vi "pathPlanningVSS.vi"(8 "error in (no error) 2":errorcluster, 9 "Line?":bool, 11 "Game in 2":refnum<class "Game.lvclass">) -> (0 "error out 2":errorcluster, 3 "Game out 2":refnum<class "Game.lvclass">)   [LabVIEW 2023, in "Game.lvclass"]
uses:
  Game.lvclass
  Game.lvclass/Game.ctl
  Read Parameters.lvclass.vi
  Parameters_class/Parameters.lvclass
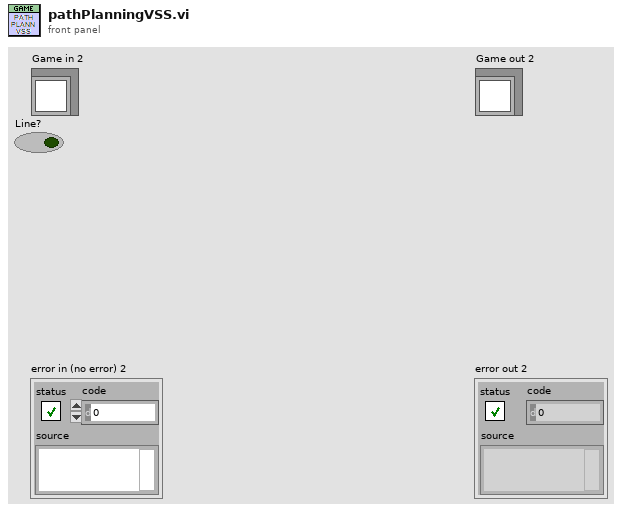
[diagram p1: front panel]
types:
  T1 = typedef "AI Input.ctl" = cluster{"our_robots":T2[], "enemy_robots":T2[], "balls":T8[], "geometry":T9, "IA Judge":T10, "Received Timestamp":timestamp, "Events":T12}
  T2 = typedef "AI Robot.ctl" = cluster{"id":u32, "function":T3, "x":dbl, "y":dbl, "orientation":dbl, "v_tangent":dbl, "v_normal":dbl, "v_ang":dbl, "kick_x":dbl, "kick_z":dbl, "dribble":bool, "Timestamp":timestamp, "estimatives":cluster{"est_v_tangent":dbl, "est_v_normal":dbl, "est_vx":dbl, "est_vy":dbl, "Pos Robot Est":dbl[]}, "dest_x_kick":dbl, "dest_y_kick":dbl, "Gap Coord":dbl[], "States":T4, "Path ":dbl[][], "Path  Smooth":dbl[][], "Dest":T5, "vx_desired":dbl, "vy_desired":dbl, "slowBehavior":bool, "VSSStates":T7}
  T3 = typedef "Functions Enum.ctl" = enum16{"2nd Striker", "Attacker", "Goalie", "Defender", "Striker", "Goto 0", "Dummy", "Kicker", "ZigZag 0", "ZigZag 1", "ZigZag 2", "ZigZag 3", "ZigZag 4", "ZigZag 5", "ZigZag 6", "ZigZag 7", "ZigZag 8", ""}
  T4 = typedef "AttackerStates.ctl" = enum16{"Pass", "GoToTangent", "BallGetting", "GoToKick", ""}
  T5 = typedef "PathDests.ctl" = T6[]
  T6 = typedef "PathDest.ctl" = cluster{"dest_x":dbl, "dest_y":dbl, "dest_orientation":dbl, "dest_vel":dbl}
  T7 = typedef "VSSAttackerStates.ctl" = enum16{"Pass", "GoToTangent", "BallGetting", "GoToKick", "Rotate anti-clockwise", "Rotate Clockwise", ""}
  T8 = typedef "AI Ball.ctl" = cluster{"x":dbl, "y":dbl, "timestamp":timestamp, "Vel_x":dbl, "Vel_y":dbl, "Pos Bola Est":dbl[], "Valid":bool}
  T9 = typedef "Field Size.ctl" = cluster{"line_width":u32, "field_length":u32, "field_width":u32, "boundary_width":u32, "referee_width":u32, "goal_width":u32, "goal_depth":u32, "goal_wall_width":u32, "center_circle_radius":u32, "defense_radius":u32, "defense_stretch":u32, "free_kick_from_defense_dist":u32, "penalty_spot_from_field_line_dist":u32, "penalty_line_from_spot_dist":u32}
  T10 = typedef "AI Judge.ctl" = cluster{"stage":string, "command":string, "our_goalie_id":dbl, "enemy_goalie_id":dbl, "command enum":T11, "Time":enum16{"Azul", "Amarelo"}}
  T11 = typedef "Command Enum.ctl" = enum16{"Halt", "Stop", "Force Start", "PKA Normal Start", "Prepare Kickoff Ally", "PKE Normal Start", "Prepare Kickoff Enemy", "Prepare Penalty Ally", "PPA Normal Start", "Prepare Penalty Enemy", "PPE Normal Start", "Direct Free Enemy", "Direct Free Ally", "Indirect Free Enemy", "Indirect Free Ally", "Timeout Enemy", "Timeout Ally", "Goal Enemy", "Goal Ally", "Ball Placement Enemy", "Ball Placement Ally", "Normal Half Time", "Extra Time Break", "Extra Half Time", "None", "Post Game"}
  T12 = typedef "Events.ctl" = cluster{"Touch":bool, "Ball out":bool, "id touch":dbl, "Ball out of \nVision":bool, "Ball inside \nGoalie area":bool, "Robot not responding":bool, "Robots responding status":dbl[], "Enemy Ball \nPossession":bool, "Pass State":bool, "id end of pass":dbl, "Kick":bool, "Id ini Possession":dbl, "Ball Possesion":bool, "Id Possesion":dbl, "Direct Kick":bool, "2nd Strk Ativo":bool}
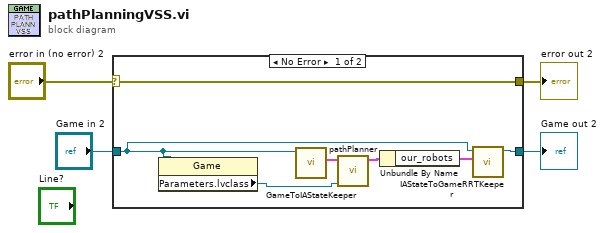
[diagram p0: block diagram]
diagram:
  n1 = case shown="No Error" "error in (no error) 2" {
    selector: "error in (no error) 2" -> [w11 w13]
    tunnel: [w11 w13] -> w3
    tunnel: [w7 w12] -> w1
    tunnel: "Game in 2" -> [w6 w12]
    frame No Error {
      n2 = property class="Game"(reference=w6) -> ("Parameters.lvclass"=w5:refnum<class "Parameters.lvclass">)  [unwired: 1 in, 2 out]
      n3 = call-dynamic "GameToIAStateKeeper.vi"("Game in"=w6) -> ("IA State out"=w9:T1)  [unwired: 8 in, 2 out]
      n4 = call "pathPlanner.vi"("Parameters.lvclass"=w5, "IA State Output in"=w9) -> ("IA State Output out"=w10:T1)  [unwired: 9 in]
      n5 = Unbundle By Name(w10) -> ("our_robots"=w8:T2[])
      n6 = call-dynamic "IAStateToGameRRTKeeper.vi"("our_robots"=w8, "Game in"=w6) -> ("Game out"=w7:refnum<class "Game.lvclass">)  [unwired: 8 in, 1 out]
    }
    frame Error {
    }
  }
  "error out 2" <- w3
  "Game out 2" <- w1
